vi "Drive Teleop Handler.vi"(10 "Call Context":T1=enum."Stop") -> ()   [LabVIEW 2023]
uses:
  swerve/Type Definitions/Data/Robot Velocities.ctl
  <vilib>/Rock Robotics/WPI/DriverStation/WPI_DriverStationDerivedRobotMode.ctl
  Drive/Implementation/Driving Mode.ctl
  <vilib>/Rock Robotics/WPI/Joystick/XBox Buttons Indexer.ctl
  ce51abe2-3967-49ec-91df-d4b8ef358bb3.vi
  20f039dc-a6f5-4e97-88ba-31848a91c715.vi
  fdc21bd4-9215-41b8-8367-bf19dde4ba27.vi
  2558f998-dd4e-4154-8f44-6f70b21d0474.vi
  <vilib>/Rock Robotics/WPI/Utilities/WPI_GetSetVariantRefNum.vi
  <vilib>/Rock Robotics/Network Tables/NT Read Number.vi
  <vilib>/Rock Robotics/Network Tables/NT Read Boolean.vi
  Framework/Robot Global Data.vi
  <vilib>/Rock Robotics/Network Tables/NT Write Boolean.vi
panel:
  out "Li4 Sees?":bool=TRUE
  in  "Deadband Info":T2={"Deadband"=0.05, "Deadband High"=1.0, "Deadband Low"=0.05}
  in  "Max Velocities":T3={"X Velocity"=15.0, "Y Velocity"=15.0, "Rotational \nVelocity"=270.0}
  in  "Sinusoidal Terms":cluster{"Max Velocity":dbl, "Frequency":dbl}
  in  "Teleop Mode":T4(ring)
  in  "Joystick Inputs":T5(array[cluster])
  in  "Send Inputs":bool
  # "reasonable terms"
  # "AprilTag ID bounds"
  # "reasonable terms"
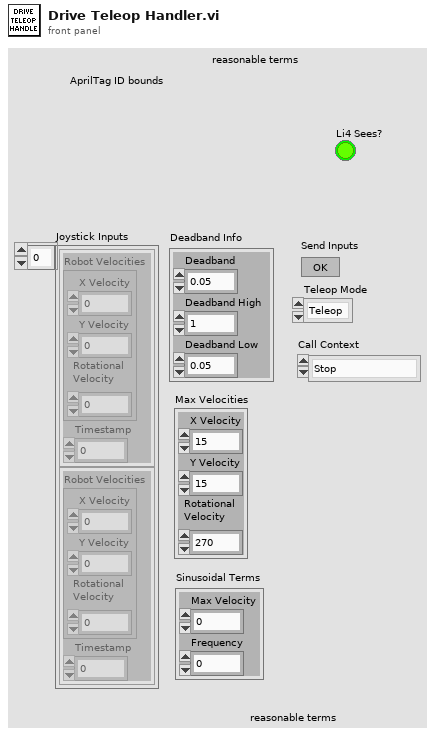
[diagram p1: front panel]
types:
  T1 = typedef "WPI_DriverStationDerivedRobotMode.ctl" = enum16{"Init", "Execute", "Stop"}
  T2 = cluster{"Deadband":dbl, "Deadband High":dbl, "Deadband Low":dbl}
  T3 = typedef "Robot Velocities.ctl" = cluster{"X Velocity":dbl, "Y Velocity":dbl, "Rotational \nVelocity":dbl}
  T4 = enum16{"Teleop", "Simulated Teleop", "Sine Velocity Profiles", "Circle Simulator"}
  T5 = cluster{"Robot Velocities":T3, "Timestamp":dbl}[]
  T6 = typedef "XBox Buttons Indexer.ctl" = enum16{"A", "B", "X", "Y", "Left Bumper", "Right Bumper", "Back", "Start", "Left Joystick", "Right Joystick"}
  T7 = typedef "Driving Mode.ctl" = enum16{"Robot Centric", "Field Centric"}
  T8 = typedef "WPI_JoystickDevRef.ctl" = cluster{"Device":T9}
  T9 = typedef "WPI_JoystickDeviceEnum.ctl" = enum16{"USB 0", "USB 1", "USB 2", "USB 3", "USB 4", "USB 5"}
  T10 = typedef "CTRE_PigeonIMU_DeviceRef.ctl" = cluster{"DeviceStatus":errorcluster, "Device Number":u8, "Type":T11, "Device ID":u32, "Handle":u64, "UsageFrame":u32, "Library Path":path}
  T11 = typedef "CTRE_PigeonIMU_ConnectionType.ctl" = u32
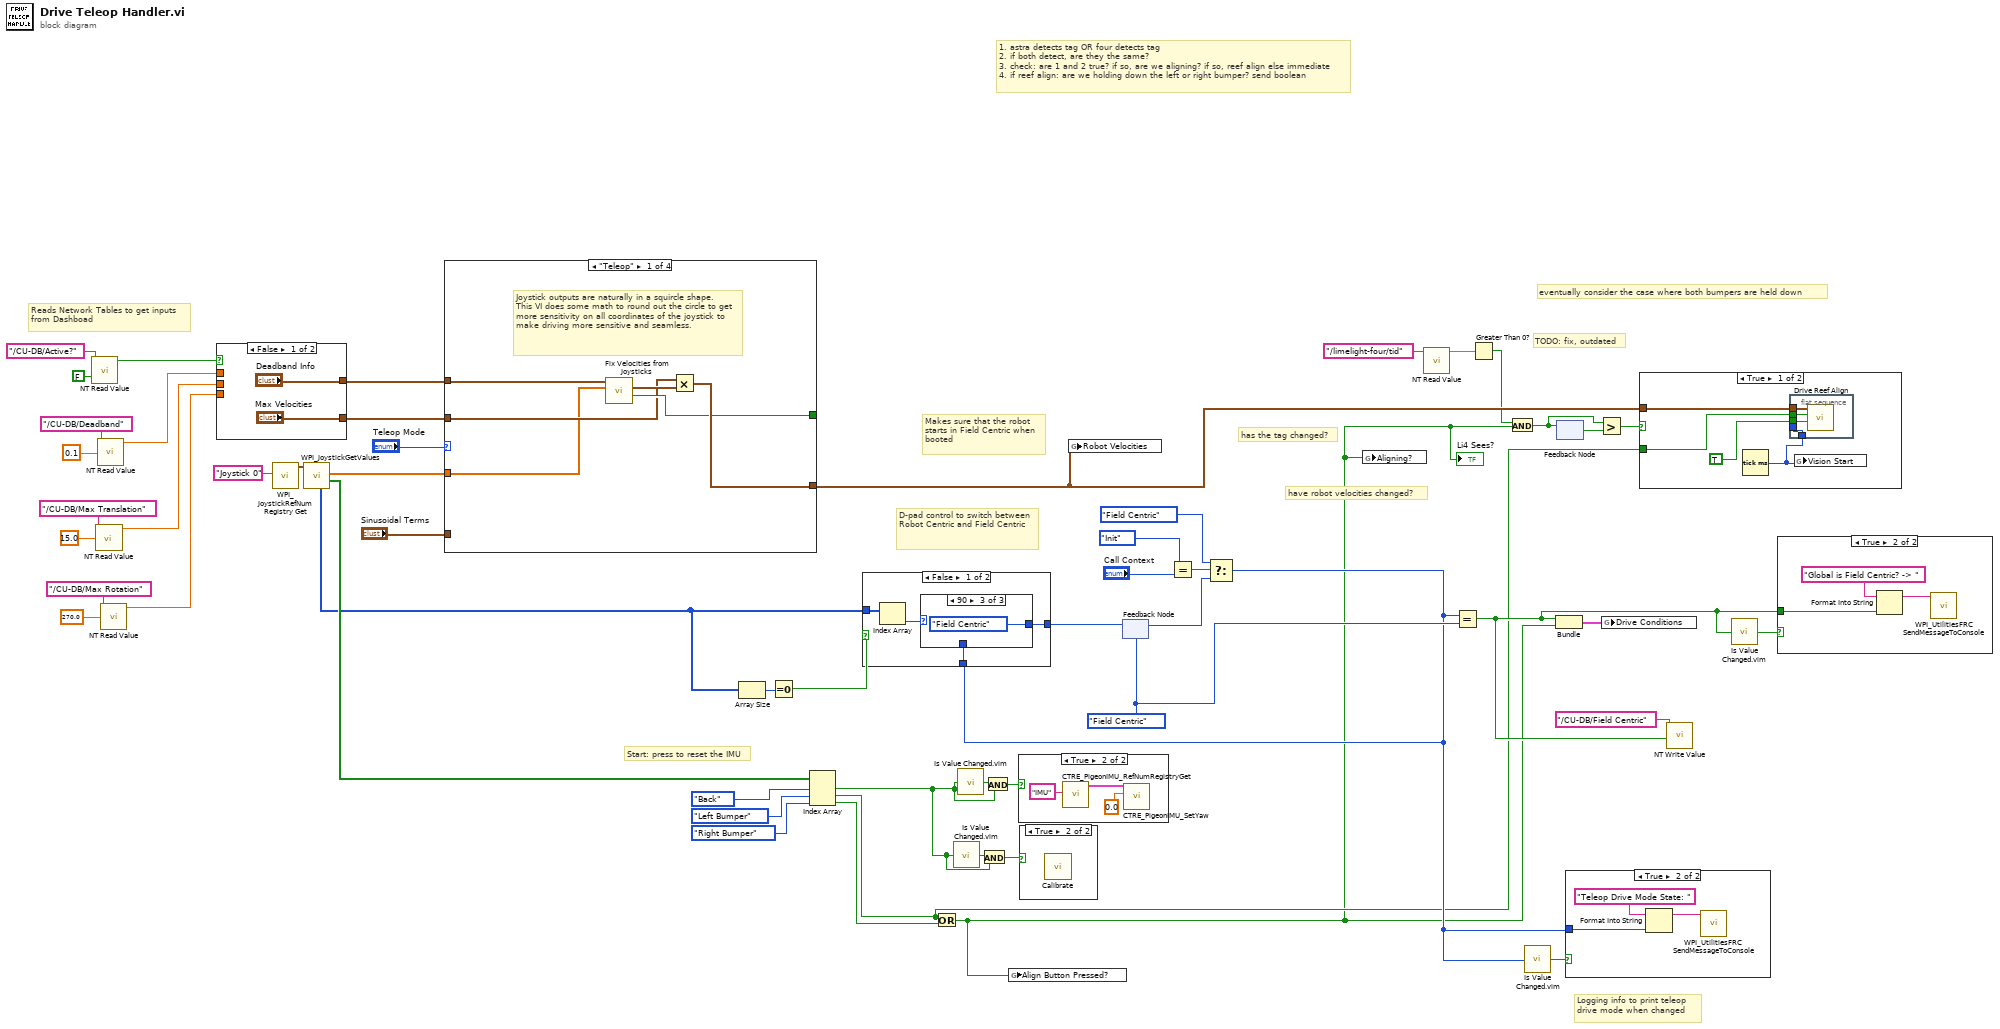
[diagram p0: block diagram]
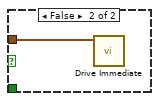
[diagram p2: hidden frame]
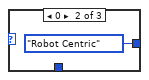
[diagram p8: hidden frame]
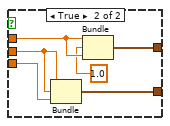
[diagram p10: hidden frame]
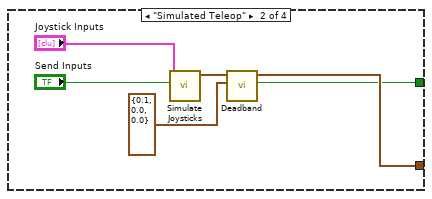
[diagram p11: hidden frame]
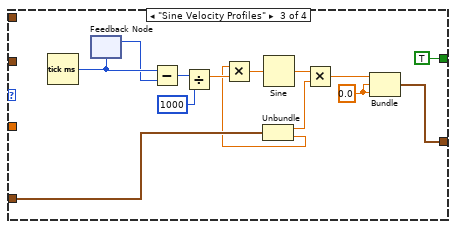
[diagram p12: hidden frame]
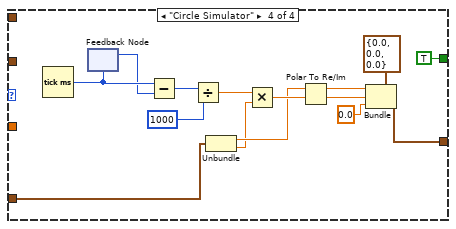
[diagram p13: hidden frame]
diagram:
  w23 = Driving_Mode."Field Centric"
  # "eventually consider the case where both bumpers are held down"
  # "1. astra detects tag OR four detects tag\n2. if both detect, are they the same?\n3. check: are 1 and 2 true? if so, are we aligning? if so, reef align else immediate\n4. if reef align: are we holding down the left or right bumper? send boolean"
  # "have robot velocities changed?"
  # "has the tag changed?"
  # "TODO: fix, outdated"
  # "Reads Network Tables to get inputs from Dashboad"
  # "Logging info to print teleop drive mode when changed"
  # "Makes sure that the robot starts in Field Centric when booted"
  # "Start: press to reset the IMU"
  # "D-pad control to switch between Robot Centric and Field Centric"
  n1 = call-poly <vilib>:"NT Read Value.vi"("default value"=FALSE ("Default Value"), "name"="/CU-DB/Active?" ("Name")) -> ("value"=w37:bool)  [unwired: 7 in, 2 out]
  n2 = call-poly <vilib>:"NT Read Value.vi"("default value"=15.0 ("Default Value"), "name"="/CU-DB/Max Translation" ("Name")) -> ("value"=w34:dbl)  [unwired: 7 in, 2 out]
  n3 = call-poly <vilib>:"NT Read Value.vi"("default value"=0.1 ("Default Value"), "name"="/CU-DB/Deadband" ("Name")) -> ("value"=w36:dbl)  [unwired: 7 in, 2 out]
  n4 = call-poly <vilib>:"NT Read Value.vi"("default value"=270.0 ("Default Value"), "name"="/CU-DB/Max Rotation" ("Name")) -> ("value"=w33:dbl)  [unwired: 7 in, 2 out]
  n5 = case shown="False" w37 {
    tunnel: w36 -> [_ w62]
    tunnel: ["Deadband Info" w60] -> w35
    tunnel: w34 -> [_ w59]
    tunnel: w33 -> [_ w58]
    tunnel: ["Max Velocities" w57] -> w32
    frame False {
    }
    frame True {
      n6 = Bundle("value"=w59, "value"=w59, "value"=w58) -> (w57:cluster{"value":dbl, "value":dbl, "value":dbl})  [unwired: 1 in]
      n7 = Bundle("value"=w62, "value"=1.0, "value"=w62) -> (w60:cluster{"value":dbl, "value":dbl, "value":dbl})  [unwired: 1 in]
    }
  }
  n8 = call <vilib>:"WPI_JoystickRefNum Registry Get.vi"("refnum name"="Joystick 0") -> ("JoystickDevRef"=w53:T8)  [unwired: 1 in, 9 out]
  n9 = call <vilib>:"WPI_JoystickGetValues.vi"("JoystickDevRef"=w53) -> ("Buttons"=w50:bool[], "Axes"=w52:dbl[], "POVs"=w30:i16[])  [unwired: 6 in, 2 out]
  n10 = case shown="\"Teleop\"" "Teleop Mode" {
    tunnel: w52 -> [w63 _ _ _]
    tunnel: [w68 w74 w79 w101] -> w8
    tunnel: "Sinusoidal Terms" -> [_ _ w78 w91]
    tunnel: w35 -> [w67 _ _ _]
    tunnel: w32 -> [w64 _ _ _]
    tunnel: [w65 w69 TRUE ("Sending Input?") TRUE ("Sending Input?")] -> _
    frame "Teleop" {
      # "Joystick outputs are naturally in a squircle shape.\nThis VI does some math to round out the circle to get more sensitivity on all coordinates of the joystick to make driving more sensitive and seamless."
      n11 = call "Fix Velocities from Joysticks.vi"("Axes"=w63, "Deadband"=w67) -> ("Sending Input?"=w65:bool, "Adjusted Robot Velocities"=w66:T3)  [unwired: 8 in]
      n12 = Multiply(x=w64, y=w66) -> (x*y=w68:T3)
    }
    frame "Simulated Teleop" {
      n13 = call "Simulate Joysticks.vi"("Send Inputs"="Send Inputs", "Joystick Inputs"="Joystick Inputs") -> ("Joystick Inputs"=w71:T3)  [unwired: 9 in]
      n14 = call "Deadband.vi"("Deadband Info"=T2 {"Deadband"=0.1, "Deadband High"=0.0, "Deadband Low"=0.0}, "Robot Velocities"=w71) -> ("Sending Input?"=w69:bool, "Adjusted Robot Velocities"=w74:T3)  [unwired: 8 in]
    }
    frame "Sine Velocity Profiles" {
      w87 = 0.0
      n15 = Tick Count (ms)() -> (millisecond timer value=w81:u32)
      n16 = feedback #1(w81) -> (w80:u32)
      n17 = feedback-in #1(w80) -> ()
      n18 = Subtract(x=w81, y=w80) -> (x-y=w85:u32)
      n19 = Divide(x=w85, y=u32 1000) -> (x/y=w83:dbl)
      n20 = Unbundle(w78) -> ("Max Velocity"=w76:dbl, "Frequency"=w77:dbl)
      n21 = Multiply(x=w77, y=w83) -> (x*y=w82:dbl)
      n22 = Sine(x=w82) -> (sin(x)=w86:dbl)
      n23 = Multiply(x=w86, y=w76) -> (x*y=w88:dbl)
      n24 = Bundle(w88, w87, w87) -> (w79:cluster{dbl, dbl, dbl})  [unwired: 1 in]
    }
    frame "Circle Simulator" {
      n25 = Tick Count (ms)() -> (millisecond timer value=w97:u32)
      n26 = feedback #2(w97) -> (w96:u32)
      n27 = feedback-in #2(w96) -> ()
      n28 = Subtract(x=w97, y=w96) -> (x-y=w99:u32)
      n29 = Divide(x=w99, y=u32 1000) -> (x/y=w93:dbl)
      n30 = Unbundle(w91) -> ("Max Velocity"=w94:dbl, "Frequency"=w92:dbl)
      n31 = Multiply(x=w93, y=w92) -> (x*y=w95:dbl)
      n32 = Polar To Re/Im(2:w95, 3:w94) -> (0:w89:dbl, 1:w90:dbl)
      n33 = Bundle(cluster=T3 {"X Velocity"=0.0, "Y Velocity"=0.0, "Rotational \nVelocity"=0.0} ("Robot Velocities (ft/s and deg/s)"), "X Velocity"=w90, "Y Velocity"=w89, "Rotational \nVelocity"=0.0 ("Rotational \nVelocity")) -> (w101:T3)
    }
  }
  n34 = Array Size(array=w30) -> (size(s)=w29:i32)
  n35 = Equal To 0?(x=w29) -> (x = 0?=w28:bool)
  n36 = Index Array(array=w50, index #1=XBox_Buttons_Indexer."Back" ("XBox Buttons"), index #2=XBox_Buttons_Indexer."Left Bumper" ("XBox Buttons"), index #3=XBox_Buttons_Indexer."Right Bumper" ("XBox Buttons")) -> (element #1=w9:bool, element #2=w10:bool, element #3=w11:bool)
  n37 = Or(x=w10, y=w11) -> (x .or. y?=w1:bool)
  "Li4 Sees?" <- w1
  n38 = call "Is Value Changed.vim"("value"=w9) -> ("changed or first call?"=w17:bool)
  n39 = call "Is Value Changed.vim"("value"=w9) -> ("changed or first call?"=w49:bool)
  n40 = And(x=w17, y=w9) -> (x .and. y?=w16:bool)
  n41 = And(x=w49, y=w9) -> (x .and. y?=w48:bool)
  n42 = global write "Robot Global Data.vi" "Align Button Pressed?"(w1) -> ()
  n43 = case shown="True" w48 {
    frame False {
    }
    frame True {
      n44 = call <vilib>:"CTRE_PigeonIMU_RefNumRegistryGet.vi"("refnum name"="IMU") -> ("PigeonIMUDevRef"=w105:T10)  [unwired: 9 in, 1 out]
      n45 = call <vilib>:"CTRE_PigeonIMU_SetYaw.vi"("Value"=0.0, "PigeonIMUDevRef"=w105) -> ()  [unwired: 8 in, 2 out]
    }
  }
  n46 = case shown="True" w16 {
    frame False {
    }
    frame True {
      n47 = call "Calibrate.vi"() -> ()  [unwired: 11 in, 1 out]
    }
  }
  n48 = global write "Robot Global Data.vi" "Robot Velocities"(w8) -> ()
  n49 = feedback #3(w23) -> (w22:T7)
  n50 = Equal?(x=WPI_DriverStationDerivedRobotMode."Init" ("y"), y="Call Context") -> (x = y?=w25:bool)
  n51 = Select(t=Driving_Mode."Field Centric" ("x"), s=w25, f=w22) -> (s? t:f=w19:T7)
  n52 = case shown="False" w28 {
    tunnel: [w109 w114] -> w51
    tunnel: w19 -> [w108 w114]
    tunnel: w30 -> [w107 _]
    frame False {
      n53 = Index Array(array=w107) -> (element=w110:i16)  [unwired: 1 in]
      n54 = case shown="90" w110 {
        tunnel: [w111 Driving_Mode."Robot Centric" Driving_Mode."Field Centric"] -> w109
        tunnel: w108 -> [w111 _ _]
        frame -1, Default {
        }
        frame 0 {
        }
        frame 90 {
        }
      }
    }
    frame True {
    }
  }
  n55 = feedback-in #3(w51) -> ()
  n56 = global write "Robot Global Data.vi" "Aligning?"(w1) -> ()
  n57 = call-poly <vilib>:"NT Read Value.vi"("name"="/limelight-four/tid") -> ("value"=w7:dbl)  [unwired: 8 in, 2 out]
  n58 = Equal?(x=w19, y=w23) -> (x = y?=w20:bool)
  n59 = Greater Than 0?(x=w7) -> (x > 0?=w5:bool)
  n60 = And(x=w5, y=w1) -> (x .and. y?=w3:bool)
  n61 = call "Is Value Changed.vim"("value"=w19) -> ("changed or first call?"=w18:bool)
  n62 = Bundle(w20, w1) -> (w12:cluster{bool, bool})  [unwired: 1 in]
  n63 = feedback #4() -> (w4:bool)  [unwired: 1 in]
  n64 = feedback-in #4(w3) -> ()
  n65 = case shown="True" w18 {
    tunnel: w19 -> [_ w115]
    frame False {
    }
    frame True {
      n66 = Format Into String(initial string="Teleop Drive Mode State: ", w115) -> (resulting string=w117:string)  [unwired: 2 in, 1 out]
      n67 = call <vilib>:"WPI_UtilitiesFRC SendMessageToConsole.vi"("Message"=w117) -> ()  [unwired: 14 in, 1 out]
    }
  }
  n68 = Greater?(x=w3, y=w4) -> (0:w2:bool)
  n69 = global write "Robot Global Data.vi" "Drive Conditions"(w12) -> ()
  n70 = case shown="True" w2 {
    tunnel: w8 -> [w120 w126]
    tunnel: w10 -> [w121 _]
    frame True {
      n71 = Tick Count (ms)() -> (millisecond timer value=w118:u32)
      n72 = flat-sequence {
        tunnel: w121 -> [w125]
        tunnel: w120 -> [w124]
        tunnel: TRUE ("Angle Align") -> [w123]
        tunnel: [w122] -> _
        tunnel: w118 -> [w122]
        frame #0 {
          n73 = call "Drive Reef Align.vi"("Angle Align"=w123, "Left Side?"=w125, "Robot Velocities"=w124) -> ()  [unwired: 8 in, 1 out]
        }
      }
      n74 = global write "Robot Global Data.vi" "Vision Start"(w118) -> ()
    }
    frame False {
      n75 = call "Drive Immediate.vi"("Robot Velocities"=w126) -> ()  [unwired: 10 in, 1 out]
    }
  }
  n76 = call-poly <vilib>:"NT Write Value.vi"("value"=w20, "name"="/CU-DB/Field Centric") -> ()  [unwired: 9 in, 1 out]
  n77 = call "Is Value Changed.vim"("value"=w20) -> ("changed or first call?"=w21:bool)
  n78 = case shown="True" w21 {
    tunnel: w20 -> [_ w128]
    frame False {
    }
    frame True {
      n79 = Format Into String(initial string="Global is Field Centric? -> ", w128) -> (resulting string=w129:string)  [unwired: 2 in, 1 out]
      n80 = call <vilib>:"WPI_UtilitiesFRC SendMessageToConsole.vi"("Message"=w129) -> ()  [unwired: 14 in, 1 out]
    }
  }
